vi "CJ Guidance().vi"() -> (3 "Guidance Library.lvlib:Constant Jerk Guidance.lvclass":refnum<class "Constant Jerk Guidance.lvclass">)   [LabVIEW 2014, in "Guidance Library.lvlib" / "Constant Jerk Guidance.lvclass"]
uses:
  Constant Jerk Guidance.lvclass
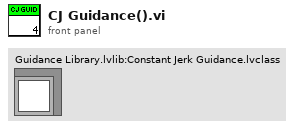
[diagram p1: front panel]
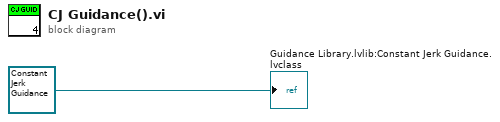
[diagram p0: block diagram]
diagram:
  "Guidance Library.lvlib:Constant Jerk Guidance.lvclass" <- refnum<class "Constant Jerk Guidance.lvclass"> refnum ("Guidance Library.lvlib:Constant Jerk Guidance.lvclass")
